vi "Change State.vi"(8 "error in (no error)":errorcluster, 10 "Target State":refnum<class "State Machine Actor.lvclass">, 11 "State Machine Actor in":refnum<class "State Machine Actor.lvclass">) -> (0 "error out":errorcluster, 3 "State Machine Actor out":refnum<class "State Machine Actor.lvclass">)   [LabVIEW 2024, in "State Machine Actor.lvlib" / "State Machine Actor.lvclass"]
doc: "-change state must be static dispatch at this level, essentially forcing all states to have the ability to nest\n-we release the notifier here so as to not force call parent in exit"
uses:
  State Machine Actor.lvclass
  C:/Program Files (x86)/National Instruments/LabVIEW 2024/vi.lib/ActorFramework/Actor/Actor.lvclass
  State Machine Actor.lvclass/State Machine Actor.ctl
  C:/Users/uspoaotto/OneDrive - Oregon Tool/Desktop/working copies/stateMachineActor/src/_State Machine Actor/_State Machine Actor/_State Machine Actor.lvclass
  C:/Users/uspoaotto/OneDrive - Oregon Tool/Desktop/working copies/stateMachineActor/src/State Machine Actor/State Machine Actor/State Machine Actor.lvclass
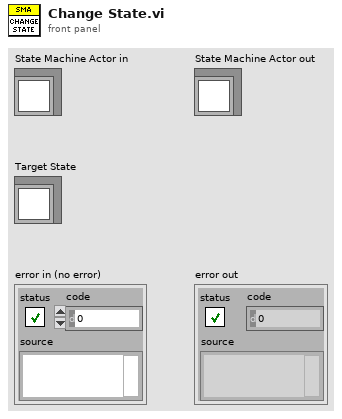
[diagram p1: front panel]
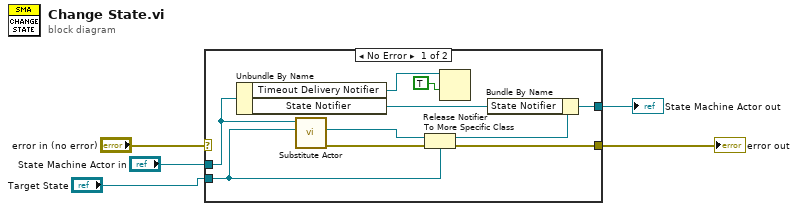
[diagram p0: block diagram]
diagram:
  n1 = case shown="No Error" "error in (no error)" {
    selector: "error in (no error)" -> [_ w17]
    tunnel: [w13 w17] -> w4
    tunnel: [w7 w16] -> w2
    tunnel: "State Machine Actor in" -> [w12 w16]
    tunnel: "Target State" -> [w6 _]
    frame No Error {
      n2 = Unbundle By Name(w12) -> ("Timeout Delivery Notifier"=w11:refnum<notifier>, "State Notifier"=w8:refnum<notifier>)
      n3 = call-dynamic "Substitute Actor.vi"("Substitute Actor in"=w6, "Current Actor"=w12) -> ("error out"=w14:errorcluster, "Substitute Actor out"=w15:refnum<class "Actor.lvclass">)  [unwired: 8 in]
      n4 = To More Specific Class(target class=w6, reference=w15, error in=w14) -> (specific class reference=w9:refnum<class "State Machine Actor.lvclass">, error out=w13:errorcluster)
      n5 = Release Notifier(notifier=w11, force destroy? (F)=TRUE) -> ()  [unwired: 1 in, 3 out]
      n6 = Bundle By Name(cluster=w9, "State Notifier"=w8) -> (w7:refnum<class "State Machine Actor.lvclass">)
    }
    frame Error {
    }
  }
  "error out" <- w4
  "State Machine Actor out" <- w2
